vi "Execute event.vi"(8 "error in (no error)":errorcluster, 9 "Event Data":variant, 10 "Button Event":T1, 11 "Vi_Button in":refnum<class "Vi_Button.lvclass">) -> (0 "error out":errorcluster, 3 "Vi_Button out":refnum<class "Vi_Button.lvclass">)   [LabVIEW 2012, in "Vi_Button.lvclass"]
doc: "Override the execute method to run the vi assocaited with this button with a vi-server call"
uses:
  Vi_Button.lvclass
  Button_Class/Type Defs/Button Events.ctl
  Vi_Button.lvclass/Vi_Button.ctl
  Button_Class/Button.lvclass
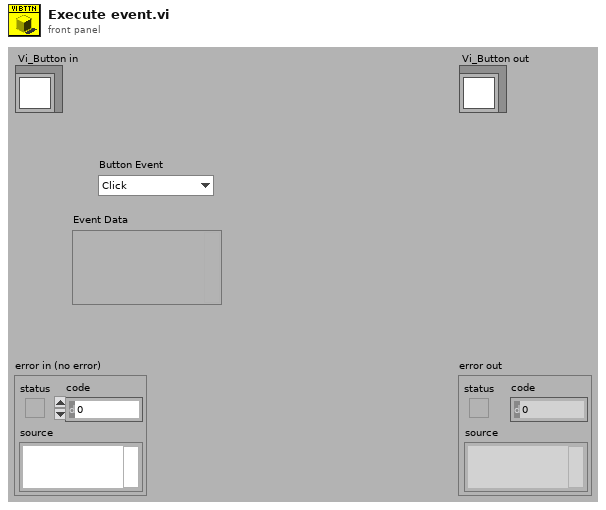
[diagram p1: front panel]
types:
  T1 = typedef "Button.lvclass/Button Events.ctl" = enum16{"Click", "Latch", "Unlatch"}
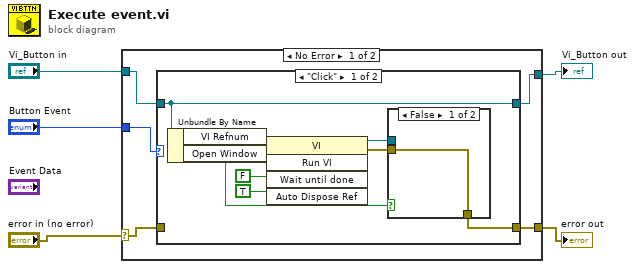
[diagram p0: block diagram]
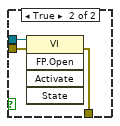
[diagram p2: hidden frame]
diagram:
  n1 = case shown="No Error" "error in (no error)" {
    selector: "error in (no error)" -> [w6 w25]
    tunnel: "Vi_Button in" -> [w8 w26]
    tunnel: "Button Event" -> [w10 _]
    tunnel: [w9 w26] -> w2
    tunnel: [w7 w25] -> w1
    frame No Error {
      n2 = case shown="\"Click\"" w10 {
        tunnel: [w11 w24] -> w9
        tunnel: w8 -> [w11 w24]
        tunnel: [w12 w23] -> w7
        tunnel: w6 -> [_ w23]
        frame "Click" {
          n3 = Unbundle By Name(w11) -> ("VI Refnum"=w18:refnum<vi>, "Open Window"=w13:bool)
          n4 = invoke class="VI" method="Run VI"(reference=w18, "Wait until done"=FALSE ("Wait Until Done"), "Auto Dispose Ref"=TRUE ("Auto Dispose Reference")) -> (reference out=w15:refnum<vi>, error out=w14:errorcluster)  [unwired: 2 in, 3 out]
          n5 = case shown="False" w13 {
            tunnel: w15 -> [_ w22]
            tunnel: w14 -> [w19 w21]
            tunnel: [w19 w20] -> w12
            frame False {
            }
            frame True {
              n6 = invoke class="VI" method="FP.Open"(reference=w22, error in=w21) -> (error out=w20:errorcluster)  [unwired: 3 in, 4 out]
            }
          }
        }
        frame "Latch", Default {
        }
      }
    }
    frame Error {
    }
  }
  "error out" <- w1
  "Vi_Button out" <- w2
